vi "FlatToRichpumploop_SetSysInfResult.vi"(5 "OutputClusterType":T1, 11 "InputCluster":T3) -> (3 "OutputCluster":T1)   [LabVIEW 2024, in "pumploop_client.lvlib"]
uses:
  pumploop_client.lvlib
  pumploop_SetSysInfResult_Flat.ctl
  pumploop_SystemInfo_Flat.ctl
  pumploop_SetSysInfResult.ctl
  pumploop_SystemInfo.ctl
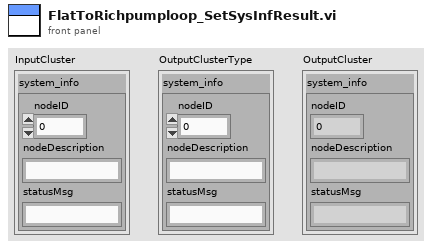
[diagram p1: front panel]
types:
  T1 = typedef "pumploop_client.lvlib/pumploop_SetSysInfResult.ctl" = cluster{"system_info":T2}
  T2 = typedef "pumploop_client.lvlib/pumploop_SystemInfo.ctl" = cluster{"nodeID":i32, "nodeDescription":string, "statusMsg":string}
  T3 = typedef "pumploop_client.lvlib/pumploop_SetSysInfResult_Flat.ctl" = cluster{"system_info":T4}
  T4 = typedef "pumploop_client.lvlib/pumploop_SystemInfo_Flat.ctl" = cluster{"nodeID":i32, "nodeDescription":string, "statusMsg":string}
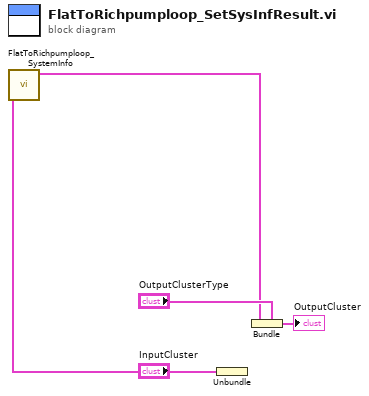
[diagram p0: block diagram]
diagram:
  n1 = Unbundle "Unbundle"("InputCluster") -> ("system_info"=w2:T4)
  n2 = call "FlatToRichpumploop_SystemInfo.vi"("InputCluster"=w2) -> ("OutputCluster"=w1:T2)  [unwired: 10 in]
  n3 = Bundle "Bundle"(cluster="OutputClusterType", "system_info"=w1) -> (→"OutputCluster":T1)
